vi "RemoveExtraLines.vi"(11 "Sensed":string[](array[string])=["", "", "", "otherNonsensedMethod 30", "", "nonsenseMethod"]) -> (3 "Output":string[](array[string]))   [LabVIEW 2014]
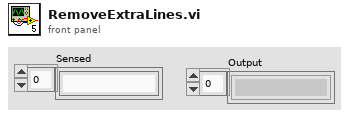
[diagram p1: front panel]
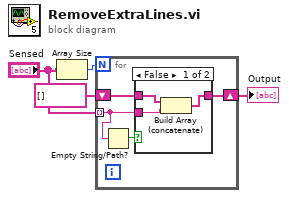
[diagram p0: block diagram]
diagram:
  n1 = Array Size(array="Sensed") -> (size(s)=w3:i32)
  n2 = for {
    N: w3 -> [_]
    tunnel: "Sensed" -> [w5] mode=indexing
    shift-right: [w6] -> w2
    shift-left: string[] [] -> [w7]
    n3 = Empty String/Path?(string/path=w5) -> (empty?=w8:bool)
    n4 = case shown="False" w8 {
      tunnel: w7 -> [w9 w12]
      tunnel: [w10 w12] -> w6
      tunnel: w5 -> [w11 _]
      frame False {
        n5 = Build Array (concatenate)(w9, w11) -> (w10:string[])
      }
      frame True {
      }
    }
  }
  "Output" <- w2
